vi "UHR-Fleezers Control (host) - 16.2.2v2.vi"() -> ()   [LabVIEW 2014] (continued)
        "Overflow (data lost)" <- TRUE ("Overflow (data lost)")
      }
    }
    n3205 = Build Array(w4581, w4580) -> (w4579:dbl[][])
    n3206 = To Double Precision Float(number=w4672) -> (double precision float=w4673:dbl[][])
    n3207 = feedback #8 "APD3"(w4368) -> (w4387:dbl[])
    n3208 = feedback #9 "APD2"(w4370) -> (w4602:dbl[])
    n3209 = feedback #10 "APD1"(w4372) -> (w4671:dbl[])
    n3210 = Build Array (concatenate)(w4387, w4368) -> (w4386:dbl[])
    n3211 = Build Array (concatenate)(w4602, w4370) -> (w4601:dbl[])
    n3212 = Build Array (concatenate)(w4671, w4372) -> (w4668:dbl[])
    n3213 = for {
      tunnel: w4370 -> [w4855] mode=indexing
      n3214 = call "Smart Buffer (DBL) 2.vi"("new element [write]"=w4855, "mode"=T26."write") -> ()  [unwired: 4 in, 6 out]
    }
    n3215 = Array Size(array=w4668) -> (size(s)=w4665:i32)
    n3216 = Array Size(array=w4372) -> (size(s)=w4667:i32)
    n3217 = Multiply(x=w4667, y="APD Ave N") -> (x*y=w4666:dbl)
    n3218 = Greater?(x=w4665, y=w4666) -> (0:w4669:bool)
    n3219 = Bundle("APD 1", "APD 2", "APD 3") -> (w4703:cluster{string, string, string})  [unwired: 1 out]
    n3220 = local read "Trap Sets"() -> (w4636:u32)
    n3221 = case shown="True" w4669 {
      tunnel: w4668 -> [w5112 w5121]
      tunnel: [w5112 w5119] -> w4643
      tunnel: w4666 -> [_ w5114]
      tunnel: w4665 -> [_ w5120]
      tunnel: w4601 -> [w5111 w5118]
      tunnel: [w5111 w5117] -> w4599
      tunnel: w4386 -> [w5110 w5116]
      tunnel: [w5110 w5113] -> w4449
      frame False {
      }
      frame True {
        n3222 = Subtract(x=w5120, y=w5114) -> (x-y=w5115:dbl)
        n3223 = Array Subset "APD3"(array=w5116, index=w5115, length=w5114) -> (w5113:dbl[])
        n3224 = Array Subset "APD2"(array=w5118, index=w5115, length=w5114) -> (w5117:dbl[])
        n3225 = Array Subset "APD1"(array=w5121, index=w5115, length=w5114) -> (w5119:dbl[])
      }
    }
    n3226 = feedback-in #8(w4449) -> ()
    n3227 = feedback-in #9(w4599) -> ()
    n3228 = feedback-in #10(w4643) -> ()
    n3229 = Cluster To Array(cluster=w4703) -> (array=w4700:string[])
    n3230 = for "APD" {
      tunnel: w4673 -> [w5368] mode=indexing
      tunnel: w4366 -> [w5375]
      tunnel: [w5371] -> w4603 mode=indexing
      tunnel: "APD Disp. Scale" -> [w5372]
      tunnel: w4700 -> [w5370] mode=indexing
      tunnel: "APD Disp. Downsample" -> [w5366]
      tunnel: [w5369] -> w4699
      workers-P: _ -> [_]
      tunnel: w4575 -> [w5365]
      n3231 = call "integrate 1D array interval - double.vi"("Ave N"=w5366, "Array In"=w5368) -> ("Array Out"=w5367:dbl[])  [unwired: 1 out]
      n3232 = Multiply(x=w5375, y=w5366) -> (x*y=w5369:dbl)
      n3233 = Divide(x=w5367, y=w5372) -> (x/y=w5373:dbl[])
      n3234 = Bundle By Name("t0"=w5365, "Y"=w5373, "dt"=w5369) -> (w5374:waveform(dbl))  [unwired: 1 out]
      n3235 = Set Waveform Attribute(5:w5370, 6:"NI_ChannelName" ("name"), 7:w5374) -> (3:w5371:waveform(dbl))  [unwired: 1 in, 2 out]
    }
    "APD Display Period (s)" <- w4699
    n3236 = Reciprocal(x=w4699) -> (1/x=→"APD Display Freq. (Hz)":dbl)
    n3237 = case "Deinterlace trap data, average down PSD" shown="2" w4636 {
      tunnel: w4548 -> [w5393 w5458]
      tunnel: [w5390 w5455] -> w4631
      tunnel: [w5393 w5457] -> w4539
      tunnel: "Detector Type" -> [w5392 w5453]
      tunnel: [w5391 w5456] -> w4630
      tunnel: [w5389 w5454] -> w4707
      frame 1, Default {
        n3238 = Divide(x=w5393, y=3276.7) -> (x/y=w5394:dbl[])
        n3239 = Decimate 1D Array(w5394) -> (w5403:dbl[], w5402:dbl[], w5401:dbl[], w5400:dbl[], w5399:dbl[], w5398:dbl[], w5397:dbl[], w5396:dbl[])
        n3240 = case shown="\"IR-QPD + PSD + FB-QPD position\"" w5392 {
          tunnel: w5403 -> [w5427 w5452]
          tunnel: w5402 -> [w5426 w5451]
          tunnel: w5401 -> [w5411 w5429]
          tunnel: w5400 -> [w5412 w5439]
          tunnel: w5399 -> [w5425 w5450]
          tunnel: w5398 -> [w5424 w5449]
          tunnel: w5397 -> [w5408 w5430]
          tunnel: w5396 -> [w5407 w5428]
          tunnel: [w5406 w5436] -> w5391
          tunnel: [w5405 w5435] -> w5390
          tunnel: [w5404 w5434] -> w5389
          frame "IR-QPD + PSD + FB-QPD", Default {
            w5404 = 0  # Channel pattern
            n3241 = Divide(x=w5427, y=w5412) -> (x/y=w5414:dbl[])
            n3242 = Divide(x=w5426, y=w5412) -> (x/y=w5413:dbl[])
            n3243 = Divide(x=w5425, y=w5408) -> (x/y=w5410:dbl[])
            n3244 = Divide(x=w5424, y=w5407) -> (x/y=w5409:dbl[])
            n3245 = Build Array(w5414, w5413, w5412, w5411, w5410, w5409, w5408, w5407) -> (w5405:dbl[][])
            n3246 = Bundle("T1 Y", "T1 X", "T1 Sum", "FB Sum", "PSD Y", "PSD X", "PSD Y Sum", "PSD X Sum") -> (w5423:T53)  [unwired: 1 out]
            n3247 = Cluster To Array(cluster=w5423) -> (array=w5406:string[])
          }
          frame "IR-QPD + PSD + FB-QPD position" {
            w5434 = 3  # Channel pattern
            n3248 = Negate(x=w5430) -> (-x=w5431:dbl[])
            n3249 = Divide(x=w5452, y=w5439) -> (x/y=w5441:dbl[])
            n3250 = Divide(x=w5451, y=w5439) -> (x/y=w5440:dbl[])
            n3251 = Divide(x=w5450, y=w5430) -> (x/y=w5438:dbl[])
            n3252 = Divide(x=w5449, y=w5431) -> (x/y=w5437:dbl[])
            n3253 = Build Array(w5441, w5440, w5439, w5428, w5429, w5438, w5437, w5430) -> (w5435:dbl[][])
            n3254 = Bundle("T1 Y", "T1 X", "T1 Sum", "FB X", "FB Sum", "PSD Y", "PSD X", "PSD Y Sum") -> (w5448:T53)  [unwired: 1 out]
            n3255 = Cluster To Array(cluster=w5448) -> (array=w5436:string[])
          }
        }
      }
      frame 2 {
        n3256 = case shown="\"IR-QPD + PSD + FB-QPD X position\", Default" w5453 {
          tunnel: w5458 -> [w5520 w5592 w5663]
          tunnel: [w5459 w5583 w5594] -> w5457
          tunnel: [w5486 w5574 w5641] -> w5456
          tunnel: [w5485 w5537 w5608] -> w5455
          tunnel: [w5479 w5572 w5639] -> w5454
          frame "IR-QPD + PSD + FB-QPD" {
            w5479 = 1  # Channel pattern
            # "time average x2 the 4th signal and the 4 psd signals (detection laser)"
            # "deinterlace 3 signals from qpd"
            n3257 = Decimate 1D Array(w5520) -> (w5519:i16[], w5518:i16[], w5484:i16[], w5517:i16[], w5507:i16[], w5505:i16[], w5504:i16[], w5502:i16[])
            n3258 = Decimate 1D Array(w5484) -> (w5483:i16[], w5482:i16[])
            n3259 = Decimate 1D Array(w5519) -> (w5516:i16[], w5488:i16[])
            n3260 = Decimate 1D Array(w5518) -> (w5515:i16[], w5513:i16[])
            n3261 = Decimate 1D Array(w5517) -> (w5514:i16[], w5512:i16[])
            n3262 = call "downsample 1D array - double.vi"("Ave N"=2.0, "Array In"=w5507) -> ("Array Out"=w5506:dbl[])  [unwired: 1 out]
            n3263 = call "downsample 1D array - double.vi"("Ave N"=2.0, "Array In"=w5505) -> ("Array Out"=w5487:dbl[])  [unwired: 1 out]
            n3264 = call "downsample 1D array - double.vi"("Ave N"=2.0, "Array In"=w5504) -> ("Array Out"=w5503:dbl[])  [unwired: 1 out]
            n3265 = call "downsample 1D array - double.vi"("Ave N"=2.0, "Array In"=w5502) -> ("Array Out"=w5501:dbl[])  [unwired: 1 out]
            n3266 = Interleave 1D Arrays(w5516, w5515, w5514, w5488, w5513, w5512, w5483, w5482, w5506, w5487, w5503, w5501) -> (w5500:dbl[])
            n3267 = Divide(x=w5500, y=3276.7) -> (x/y=w5499:dbl[])
            n3268 = Decimate 1D Array(w5499) -> (w5498:dbl[], w5497:dbl[], w5496:dbl[], w5495:dbl[], w5494:dbl[], w5493:dbl[], w5481:dbl[], w5480:dbl[], w5492:dbl[], w5491:dbl[], w5490:dbl[], w5489:dbl[])
            n3269 = Divide(x=w5498, y=w5496) -> (x/y=w5466:dbl[])
            n3270 = Divide(x=w5497, y=w5496) -> (x/y=w5465:dbl[])
            n3271 = Divide(x=w5495, y=w5493) -> (x/y=w5464:dbl[])
            n3272 = Divide(x=w5494, y=w5493) -> (x/y=w5463:dbl[])
            n3273 = Divide(x=w5492, y=w5490) -> (x/y=w5462:dbl[])
            n3274 = Divide(x=w5491, y=w5489) -> (x/y=w5461:dbl[])
            n3275 = Build Array(w5466, w5465, w5496, w5464, w5463, w5493, w5481, w5480, w5462, w5461, w5490, w5489) -> (w5485:dbl[][])
            n3276 = Bundle("T1 Y", "T1 X", "T1 Sum", "T2 Y", "T2 X", "T2 Sum", "T1 FB Sum", "T2 FB Sum", "PSD Y", "PSD X", "PSD Y Sum", "PSD X Sum") -> (w5467:T54)  [unwired: 1 out]
            n3277 = To Word Integer(number=w5500) -> (16bit integer=w5459:i16[])
            n3278 = Cluster To Array(cluster=w5467) -> (array=w5486:string[])
          }
          frame "IR-QPD + PSD + FB-QPD X position", Default {
            w5572 = 2  # Channel pattern
            # "time average x2 the 3 psd signals (detection laser)"
            # "deinterlace 3 signals from qpds"
            n3279 = Decimate 1D Array(w5592) -> (w5591:i16[], w5590:i16[], w5573:i16[], w5589:i16[], w5535:i16[], w5532:i16[], w5529:i16[], w5560:i16[])
            n3280 = Select(t=i16 -1, s="Flip X Sign", f=i16 1) -> (s? t:f=w5525:i16)
            n3281 = Multiply(x=w5590, y=w5525) -> (x*y=w5526:i16[])
            n3282 = Decimate 1D Array(w5573) -> (w5558:i16[], w5556:i16[])
            n3283 = Decimate 1D Array(w5591) -> (w5588:i16[], w5575:i16[])
            n3284 = Decimate 1D Array(w5526) -> (w5587:i16[], w5585:i16[])
            n3285 = Decimate 1D Array(w5589) -> (w5586:i16[], w5584:i16[])
            n3286 = Decimate 1D Array(w5560) -> (w5559:i16[], w5557:i16[])
            n3287 = call "downsample 1D array - I16.vi"("Ave N"=2.0, "Array In"=w5535) -> ("Array Out"=w5533:i16[])  [unwired: 1 in]
            n3288 = call "downsample 1D array - I16.vi"("Ave N"=2.0, "Array In"=w5529) -> ("Array Out"=w5527:i16[])  [unwired: 1 in]
            n3289 = call "downsample 1D array - I16.vi"("Ave N"=2.0, "Array In"=w5532) -> ("Array Out"=w5530:i16[])  [unwired: 1 in]
            n3290 = Interleave 1D Arrays(w5588, w5587, w5586, w5575, w5585, w5584, w5559, w5558, w5557, w5556, w5533, w5530, w5527) -> (w5583:i16[])
            n3291 = Divide(x=w5583, y=3276.7) -> (x/y=w5582:dbl[])
            n3292 = Decimate 1D Array(w5582) -> (w5581:dbl[], w5580:dbl[], w5579:dbl[], w5578:dbl[], w5577:dbl[], w5576:dbl[], w5548:dbl[], w5546:dbl[], w5545:dbl[], w5543:dbl[], w5542:dbl[], w5541:dbl[], w5538:dbl[])
            n3293 = Negate(x=w5538) -> (-x=w5536:dbl[])
            n3294 = Divide(x=w5542, y=w5538) -> (x/y=w5540:dbl[])
            n3295 = Divide(x=w5541, y=w5536) -> (x/y=w5539:dbl[])
            n3296 = Divide(x=w5581, y=w5579) -> (x/y=w5564:dbl[])
            n3297 = Divide(x=w5580, y=w5579) -> (x/y=w5563:dbl[])
            n3298 = Divide(x=w5578, y=w5576) -> (x/y=w5562:dbl[])
            n3299 = Divide(x=w5577, y=w5576) -> (x/y=w5561:dbl[])
            n3300 = Divide(x=w5548, y=w5546) -> (x/y=w5547:dbl[])
            n3301 = Divide(x=w5545, y=w5543) -> (x/y=w5544:dbl[])
            n3302 = Build Array(w5564, w5563, w5579, w5562, w5561, w5576, w5547, w5546, w5544, w5543, w5540, w5539, w5538) -> (w5537:dbl[][])
            n3303 = Bundle("T1 Y", "T1 X", "T1 Sum", "T2 Y", "T2 X", "T2 Sum", "T1 FB X", "T1 FB Sum", "T2 FB X", "T2 FB Sum", "PSD Y", "PSD X", "PSD Y Sum") -> (w5565:T55)  [unwired: 1 out]
            n3304 = Cluster To Array(cluster=w5565) -> (array=w5574:string[])
          }
          frame "IR-QPD + PSD + FB-QPD XY positions" {
            w5639 = 4  # Channel pattern
            # "time average x2 the 3 psd signals (detection laser)"
            # "deinterlace 3 signals from qpds"
            n3305 = Decimate 1D Array(w5663) -> (w5662:i16[], w5661:i16[], w5640:i16[], w5660:i16[], w5606:i16[], w5652:i16[], w5651:i16[], w5628:i16[])
            n3306 = Decimate 1D Array "Feedback Sum"(w5640) -> (w5624:i16[], w5622:i16[])
            n3307 = Decimate 1D Array "QPD Y"(w5662) -> (w5659:i16[], w5642:i16[])
            n3308 = Decimate 1D Array "QPD X"(w5661) -> (w5658:i16[], w5656:i16[])
            n3309 = Decimate 1D Array "Feedback Y"(w5606) -> (w5605:i16[], w5604:i16[])
            n3310 = Decimate 1D Array "QPD Sum"(w5660) -> (w5657:i16[], w5655:i16[])
            n3311 = Decimate 1D Array "Feedback X"(w5628) -> (w5625:i16[], w5623:i16[])
            n3312 = call "downsample 1D array - double.vi"("Ave N"=2.0, "Array In"=w5652) -> ("Array Out"=w5627:dbl[])  [unwired: 1 out]
            n3313 = call "downsample 1D array - double.vi"("Ave N"=2.0, "Array In"=w5651) -> ("Array Out"=w5626:dbl[])  [unwired: 1 out]
            n3314 = Interleave 1D Arrays(w5659, w5658, w5657, w5642, w5656, w5655, w5605, w5625, w5624, w5604, w5623, w5622, w5627, w5626) -> (w5650:dbl[])
            n3315 = Divide(x=w5650, y=3276.7) -> (x/y=w5649:dbl[])
            n3316 = Decimate 1D Array(w5649) -> (w5648:dbl[], w5647:dbl[], w5646:dbl[], w5645:dbl[], w5644:dbl[], w5643:dbl[], w5601:dbl[], w5615:dbl[], w5599:dbl[], w5600:dbl[], w5613:dbl[], w5597:dbl[], w5611:dbl[], w5609:dbl[])
            n3317 = Negate(x=w5609) -> (-x=w5607:dbl[])
            n3318 = Divide(x=w5611, y=w5607) -> (x/y=w5610:dbl[])
            n3319 = Divide(x=w5600, y=w5597) -> (x/y=w5596:dbl[])
            n3320 = Divide(x=w5601, y=w5599) -> (x/y=w5598:dbl[])
            n3321 = Divide(x=w5648, y=w5646) -> (x/y=w5632:dbl[])
            n3322 = Divide(x=w5647, y=w5646) -> (x/y=w5631:dbl[])
            n3323 = Divide(x=w5645, y=w5643) -> (x/y=w5630:dbl[])
            n3324 = Divide(x=w5644, y=w5643) -> (x/y=w5629:dbl[])
            n3325 = Divide(x=w5615, y=w5599) -> (x/y=w5614:dbl[])
            n3326 = Divide(x=w5613, y=w5597) -> (x/y=w5612:dbl[])
            n3327 = Build Array(w5632, w5631, w5646, w5630, w5629, w5643, w5598, w5614, w5599, w5596, w5612, w5597, w5610, w5609) -> (w5608:dbl[][])
            n3328 = Bundle("T1 Y", "T1 X", "T1 Sum", "T2 Y", "T2 X", "T2 Sum", "T1 FB Y", "T1 FB X", "T1 FB Sum", "T2 FB Y", "T2 FB X", "T2 FB Sum", "PSD X", "PSD Y Sum") -> (w5595:T56)  [unwired: 1 out]
            n3329 = To Word Integer(number=w5650) -> (16bit integer=w5594:i16[])
            n3330 = Cluster To Array(cluster=w5595) -> (array=w5641:string[])
          }
        }
      }
    }
    "AI labels" <- w4630
    n3331 = Array Size(array=w4643) -> (size(s)=w4664:i32)
    n3332 = call <vilib>:"Std Deviation and Variance.vi"("X"=w4599) -> ("standard deviation"=w4598:dbl)  [unwired: 1 in, 2 out]
    n3333 = Add Array Elements(numeric array=w4599) -> (sum=w4600:dbl)
    n3334 = Add Array Elements(numeric array=w4643) -> (sum=w4674:dbl)
    n3335 = call <vilib>:"Std Deviation and Variance.vi"("X"=w4643) -> ("standard deviation"=w4642:dbl)  [unwired: 1 in, 2 out]
    n3336 = Divide(x=w4598, y=w4366) -> (x/y=w4595:dbl)
    "Rate sigma (Hz) 2" <- w4595
    n3337 = Multiply(x=w4366, y=w4664) -> (x*y=w4450:dbl)
    "Int. Time (s)" <- w4450
    n3338 = Divide(x=w4600, y=w4450) -> (x/y=w4596:dbl)
    "APD 2 Rate (Hz)" <- w4596
    n3339 = Multiply(x="APD Disp. Scale", y=w4603) -> (x*y=w4609:waveform(dbl)[])
    n3340 = Divide(x=w4674, y=w4450) -> (x/y=w4640:dbl)
    "APD 1 Rate (Hz)" <- w4640
    n3341 = Divide(x=w4642, y=w4366) -> (x/y=w4641:dbl)
    "Rate sigma (Hz)" <- w4641
    n3342 = Divide(x=w4595, y=w4596) -> (x/y=→"Sigma/Mean 2":dbl)
    n3343 = Multiply(x="APD Disp. Downsample", y=w4366) -> (x*y=w4606:dbl)
    n3344 = Divide(x=w4641, y=w4640) -> (x/y=→"Sigma/Mean":dbl)
    n3345 = Divide(x=w4609, y=w4606) -> (x/y=w4441:waveform(dbl)[])
    n3346 = Index Array(array=w4441, index=0) -> (element=w4592:waveform(dbl))
    n3347 = Index Array(array=w4441, index=1) -> (element=w4590:waveform(dbl))
    n3348 = Index Array(array=w4441, index=2) -> (element=w4443:waveform(dbl))
    n3349 = Subtract(x=w4592, y="APD 1 Offset") -> (x-y=w4588:waveform(dbl))
    n3350 = Subtract(x=w4590, y="APD 2 Offset") -> (x-y=w4587:waveform(dbl))
    n3351 = Subtract(x=w4443, y="APD 3 Offset") -> (x-y=w4440:waveform(dbl))
    n3352 = Add Array Elements(numeric array=w4449) -> (sum=w4452:dbl)
    n3353 = call <vilib>:"Std Deviation and Variance.vi"("X"=w4449) -> ("standard deviation"=w4451:dbl)  [unwired: 1 in, 2 out]
    n3354 = Build Array(w4588, w4587, w4440) -> (→"APD Chart":waveform(dbl)[])
    n3355 = Divide(x=w4452, y=w4450) -> (x/y=w4447:dbl)
    "APD 3 Rate (Hz)" <- w4447
    n3356 = Divide(x=w4451, y=w4366) -> (x/y=w4448:dbl)
    "Rate sigma (Hz) 3" <- w4448
    n3357 = Divide(x=w4448, y=w4447) -> (x/y=→"Sigma/Mean 3":dbl)
    n3358 = local read "Data Period (s)"() -> (w4498:dbl)
    n3359 = local read "BD 1 Frequency 2 (MHz)"() -> (w4531:dbl)
    n3360 = local read "BD 1 Frequency 1 (MHz)"() -> (w4532:dbl)
    n3361 = Decimate 1D Array(w4539) -> (w4563:i16[], w4562:i16[], w4560:i16[], w4559:i16[])  [unwired: 9 out]
    n3362 = Multiply(x=w4498, y="Trap Pos. Disp. Downsample") -> (x*y=w4496:dbl)
    n3363 = Divide(x=w4563, y=w4562) -> (x/y=w4564:dbl[])
    n3364 = Divide(x=w4560, y=w4559) -> (x/y=w4561:dbl[])
    n3365 = local read "AOM X Cal (nm/MHz)"() -> (w4529:dbl)
    n3366 = Split 1D Array(array=w4564, index="N El. to Ave.") -> (second subarray=w4567:dbl[])  [unwired: 1 out]
    n3367 = Split 1D Array(array=w4561, index="N El. to Ave.") -> (second subarray=w4566:dbl[])  [unwired: 1 out]
    n3368 = Multiply(x=w4498, y="Trap Disp. Downsample") -> (x*y=w4577:dbl)
    "Display Period (s)" <- w4577
    n3369 = for "Trap AI" {
      tunnel: [w5388] -> w4410 mode=indexing
      tunnel: w4575 -> [w5379]
      tunnel: "Trap Disp. Downsample" -> [w5386]
      tunnel: w4631 -> [w5384] mode=indexing
      tunnel: w4498 -> [w5383]
      tunnel: w4630 -> [w5382] mode=indexing
      tunnel: [w5381] -> w4605 mode=indexing
      tunnel: w4577 -> [w5380]
      workers-P: _ -> [_]
      n3370 = Bundle By Name("Y"=w5384, "dt"=w5383) -> (w5385:waveform(dbl))  [unwired: 1 out]
      n3371 = Set Waveform Attribute(5:w5382, 6:"NI_ChannelName" ("name"), 7:w5385) -> (3:w5381:waveform(dbl))  [unwired: 1 in, 2 out]
      n3372 = call "downsample 1D array - double.vi"("Ave N"=w5386, "Array In"=w5384) -> ("Array Out"=w5387:dbl[])  [unwired: 1 out]
      n3373 = Bundle By Name(cluster=w5381, "t0"=w5379, "Y"=w5387, "dt"=w5380) -> (w5388:waveform(dbl))
    }
    n3374 = Bundle("BD 1 Frequency 1 (MHz)"=w4532, "BD 1 Frequency 2 (MHz)"=w4531) -> (w4533:T57)  [unwired: 1 out]
    n3375 = call-poly <vilib>:"Mean.vi"("X"=w4566) -> ("mean"=w4554:dbl)  [unwired: 1 out]
    n3376 = call-poly <vilib>:"Mean.vi"("X"=w4567) -> ("mean"=w4555:dbl)  [unwired: 1 out]
    n3377 = Reciprocal(x=w4577) -> (1/x=→"Trap Disp. Freq. (Hz)":dbl)
    n3378 = Cluster To Array(cluster=w4533) -> (array=w4530:dbl[])
    n3379 = local read "Trap X AI1 (DMA)"() -> (w4565:T15)
    n3380 = local read "Data points/scans (MCL)"() -> (w4684:dbl)
    n3381 = To Fixed-Point(number=w4554) -> (fixed-point=w4552:fxp<+/-,16,1>)  [unwired: 1 in]
    n3382 = To Fixed-Point(number=w4555) -> (fixed-point=w4553:fxp<+/-,16,1>)  [unwired: 1 in]
    n3383 = Bundle("Trap 1 Pos.", "Trap 2 Pos.") -> (w4574:cluster{string, string})  [unwired: 1 out]
    n3384 = Bundle By Name(cluster=w4565, "Set 1"=w4553, "Set 2"=w4552) -> (→"Trap X AI1 (DMA)":T15)
    n3385 = Cluster To Array(cluster=w4574) -> (array=w4571:string[])
    n3386 = Unbundle(w4438) -> ("Array Out"=w4439:dbl[])  [unwired: 2 out]
    n3387 = Select(t=-1.0, s="Negate Y Axis", f=1.0) -> (s? t:f=w4515:dbl)
    n3388 = for "Trap Position" {
      tunnel: w4579 -> [w5026] mode=indexing
      tunnel: "Trap Pos. Disp. Downsample" -> [w5025]
      tunnel: w4496 -> [w5023]
      tunnel: w4575 -> [w5022]
      tunnel: w4571 -> [w5020] mode=indexing
      tunnel: [w5019] -> w4485 mode=indexing
      tunnel: w4530 -> [w5017] mode=indexing
      tunnel: w4529 -> [w5015]
      tunnel: w4515 -> [w5014]
      n3389 = call "downsample 1D array - double.vi"("Ave N"=w5025, "Array In"=w5026) -> ("Array Out"=w5024:dbl[])  [unwired: 1 out]
      n3390 = Subtract(x=w5024, y=w5017) -> (x-y=w5018:dbl[])
      n3391 = Multiply(x=w5015, y=w5018) -> (x*y=w5016:dbl[])
      n3392 = Multiply(x=w5014, y=w5016) -> (x*y=w5013:dbl[])
      n3393 = Bundle By Name("Y"=w5013, "dt"=w5023, "t0"=w5022) -> (w5021:waveform(dbl))  [unwired: 1 out]
      n3394 = Set Waveform Attribute(5:w5020, 6:"NI_ChannelName" ("name"), 7:w5021) -> (3:w5019:waveform(dbl))  [unwired: 1 in, 2 out]
    }
    n3395 = To Double Precision Float(number=w4439) -> (double precision float=w4628:dbl[])
    n3396 = local read "Display Period (s)"() -> (w4619:dbl)
    n3397 = Increment(x=w4684) -> (x+1=w4685:dbl)
    n3398 = Index Array(array=w4485, index=0) -> (element=w4489:waveform(dbl))
    n3399 = Index Array(array=w4485, index=1) -> (element=w4484:waveform(dbl))
    n3400 = feedback #11(w4685) -> (w4688:dbl)
    n3401 = Select(t=0, s=w4675, f=w4688) -> (s? t:f=w4681:dbl)
    n3402 = Array Size(array=w4628) -> (size(s)=w4687:i32)
    n3403 = Add(x=w4687, y=w4681) -> (x+y=w4682:dbl)
    n3404 = Unbundle By Name(w4489) -> ("Y"=w4490:dbl[])
    n3405 = Divide(x="Bead Sep. Int. Time (s)", y=w4619) -> (x/y=w4525:dbl)
    n3406 = Add(x=w4490, y="FB Trap Pos Offset") -> (x+y=w4488:dbl[])
    "T1 x pos data" <- w4488
    n3407 = Greater?(x=w4682, y=w4684) -> (0:w4683:bool)
    n3408 = feedback #12(w4488) -> (w4527:dbl[])
    n3409 = Build Array (concatenate)(w4488, w4527) -> (w4526:dbl[])
    n3410 = Bundle By Name(cluster=w4489, "Y"=w4488) -> (w4487:waveform(dbl))
    n3411 = Select(t=w4681, s=w4683, f=w4682) -> (s? t:f=w4680:dbl)
    n3412 = feedback-in #11(w4680) -> ()
    n3413 = local read "MCL Scanning"() -> (w4678:bool)
    n3414 = Bundle(w4487, w4484) -> (w4483:cluster{waveform(dbl), waveform(dbl)})  [unwired: 1 out]
    n3415 = Index Array(array=w4410, index="index 1") -> (element=w4432:waveform(dbl))
    n3416 = Index Array(array=w4410, index="index 2") -> (element=w4436:waveform(dbl))
    n3417 = Split 1D Array(array=w4526, index=w4525) -> (first subarray=w4519:dbl[])  [unwired: 1 out]
    n3418 = feedback-in #12(w4519) -> ()
    n3419 = Unbundle By Name(w4432) -> ("Y"=w4431:dbl[])
    n3420 = Unbundle By Name(w4436) -> ("Y"=w4435:dbl[])
    n3421 = Not(x=w4683) -> (.not. x?=w4677:bool)
    n3422 = Cluster To Array(cluster=w4483) -> (array=w4462:waveform(dbl)[])
    "Trap Positions" <- w4462
    n3423 = call-poly <vilib>:"Mean.vi"("X"=w4519) -> ("mean"=w4518:dbl)  [unwired: 1 out]
    "Mean T1 Position (nm)" <- w4518
    n3424 = Subtract(x=w4519, y=w4518) -> (x-y=w4524:dbl[])
    n3425 = Square(x=w4524) -> (x^2=w4523:dbl[])
    n3426 = And(x=w4677, y=w4678) -> (x .and. y?=w4679:bool)
    n3427 = call-poly <vilib>:"Mean.vi"("X"=w4523) -> ("mean"=w4522:dbl)  [unwired: 1 out]
    n3428 = call-poly <vilib>:"Mean.vi"("X"=w4431) -> ("mean"=→"Trap 1 sum mean":dbl)  [unwired: 1 out]
    n3429 = call-poly <vilib>:"Mean.vi"("X"=w4435) -> ("mean"=→"Trap 2 sum mean":dbl)  [unwired: 1 out]
    n3430 = Square Root(x=w4522) -> (sqrt(x)=w4521:dbl)
    n3431 = Or(x=w4679, y=w4675) -> (x .or. y?=w4676:bool)
    n3432 = Build Array (concatenate)(w4603, w4410) -> (w4390:waveform(dbl)[])
    "All Signals" <- w4390
    n3433 = Equal?(x="Tab Control 6", y=T45."High Res Display") -> (x = y?=w4632:bool)
    n3434 = case shown="False" "X or Y?" {
      tunnel: w4410 -> [w4845 w4851]
      tunnel: [w4846 w4850] -> w4405
      tunnel: [w4844 w4849] -> w4402
      frame False {
        n3435 = Index Array(array=w4845, index=0) -> (element=w4846:waveform(dbl))
        n3436 = Index Array(array=w4845, index=3) -> (element=w4844:waveform(dbl))
      }
      frame True {
        n3437 = Index Array(array=w4851, index=1) -> (element=w4850:waveform(dbl))
        n3438 = Index Array(array=w4851, index=4) -> (element=w4849:waveform(dbl))
      }
    }
    n3439 = Multiply(x=10.0, y=w4521) -> (x*y=→"Trap 1 Position RMS (A)":dbl)
    n3440 = case "For displaying the high resolution display (no downsampling)" shown="True" w4632 {
      tunnel: w4605 -> [_ w5046]
      frame False {
      }
      frame True {
        n3441 = Index Array(array=w5046, index="High Res. Display") -> (element=w5047:waveform(dbl))
        n3442 = call <vilib>:"Std Deviation and Variance.vi"("X"=w5047) -> ("mean"=w5054:dbl, "standard deviation"=w5059:dbl)  [unwired: 1 in, 1 out]
        "Mean Intensity" <- w5054
        "Sigma" <- w5059
        n3443 = Subtract(x=w5047, y=w5054) -> (x-y=w5053:waveform(dbl))
        n3444 = Select(t=w5053, s="Subtract mean", f=w5047) -> (s? t:f=→"1 Channel":waveform(dbl))
        n3445 = Divide(x=w5059, y=w5054) -> (x/y=→"Sigma/Mean":dbl)
        n3446 = feedback #13(1) -> (w5048:i32)
        n3447 = Greater Or Equal?(x=w5048, y="Slow mean N ave.") -> (x >= y?=w5061:bool)
        n3448 = Increment(x=w5048) -> (x+1=w5063:i32)
        n3449 = Select(t=1, s=w5061, f=w5063) -> (s? t:f=w5050:i32)
        n3450 = feedback-in #13(w5050) -> ()
        n3451 = feedback #14() -> (w5051:waveform(dbl))  [unwired: 1 out]
        n3452 = case shown="Default" w5048 {
          tunnel: [w5066 w5069] -> w5052
          tunnel: w5051 -> [w5068 _]
          tunnel: w5047 -> [w5067 w5069]
          frame Default {
            n3453 = call-poly <vilib>:"Append Waveforms.vi"("waveform B"=w5067, "waveform A"=w5068) -> ("waveform out"=w5066:waveform(dbl))  [unwired: 1 in, 8 out]
          }
          frame 1 {
          }
        }
        n3454 = feedback-in #14(w5052) -> ()
        n3455 = case shown="True" w5061 {
          tunnel: w5052 -> [_ w5065]
          frame False {
          }
          frame True {
            n3456 = call-poly <vilib>:"Mean.vi"("X"=w5065) -> ("mean"=→"Slow mean":dbl)  [unwired: 1 out]
          }
        }
      }
    }
    n3457 = case "For plotting results of scanning MCL (fluorescence and detection laser images)" shown="True" w4676 {
      tunnel: w4675 -> [_ w5129]
      tunnel: w4684 -> [_ _]
      tunnel: w4605 -> [_ w5256]
      tunnel: w4585 -> [_ w5164]
      tunnel: w4438 -> [_ w5135]
      frame False {
      }
      frame True {
        w5145 = u32 0 items=["Horizontal", "Vertical", "Central", "1st Diagonal", "2nd Diagonal"] ("Type of Symmetry")
        w5171 = u32 0 items=["Horizontal", "Vertical", "Central", "1st Diagonal", "2nd Diagonal"] ("Type of Symmetry")
        w5195 = u32 0 items=["Horizontal", "Vertical", "Central", "1st Diagonal", "2nd Diagonal"] ("Type of Symmetry")
        w5198 = u32 0 items=["Horizontal", "Vertical", "Central", "1st Diagonal", "2nd Diagonal"] ("Type of Symmetry")
        w5227 = u32 0 items=["Horizontal", "Vertical", "Central", "1st Diagonal", "2nd Diagonal"] ("Type of Symmetry")
        n3458 = Unbundle(w5135) -> ("Array Out"=w5134:dbl[], "Array Out"=w5132:dbl[], "Array Out"=w5130:dbl[])
        n3459 = To Double Precision Float(number=w5134) -> (double precision float=w5133:dbl[])
        n3460 = To Double Precision Float(number=w5132) -> (double precision float=w5131:dbl[])
        n3461 = To Double Precision Float(number=w5130) -> (double precision float=w5123:dbl[])
        n3462 = Index Array(array=w5256, index=10) -> (element=w5262:waveform(dbl))
        n3463 = Index Array(array=w5256, index=11) -> (element=w5259:waveform(dbl))
        n3464 = local read "Cycles/step (MCL)"() -> (w5212:u64)
        n3465 = Index Array(array=w5256, index="Channel") -> (element=w5258:waveform(dbl))
        n3466 = Unbundle(w5164) -> ("New Image"=w5163:T2, "New Image"=w5162:T2, "New Image"=w5136:T2, "New Image"=w5137:T2, "New Image"=w5138:T2)
        n3467 = local read "Scan steps (MCL)"() -> (w5125:u64)
        n3468 = Unbundle By Name(w5262) -> ("Y"=w5214:dbl[])
        n3469 = Unbundle By Name(w5259) -> ("Y"=w5216:dbl[])
        n3470 = local read "Scan lines (y)"() -> (w5126:u64)
        n3471 = local read "N APD Samp/step"() -> (w5128:dbl)
        n3472 = Unbundle By Name(w5258) -> ("Y"=w5221:dbl[])
        n3473 = call "downsample 1D array - double.vi"("Ave N"=w5212, "Array In"=w5214) -> ("Array Out"=w5213:dbl[])  [unwired: 1 out]
        n3474 = call "downsample 1D array - double.vi"("Ave N"=w5212, "Array In"=w5216) -> ("Array Out"=w5215:dbl[])  [unwired: 1 out]
        n3475 = call "downsample 1D array - double.vi"("Ave N"=w5212, "Array In"=w5221) -> ("Array Out"=w5220:dbl[])  [unwired: 1 out]
        n3476 = Multiply(x=w5125, y=u64 2) -> (x*y=w5127:u64)
        n3477 = feedback #15(w5131) -> (w5189:dbl[])
        n3478 = Build Array (concatenate)(w5189, w5131) -> (w5188:dbl[])
        n3479 = feedback #16(w5123) -> (w5124:dbl[])
        n3480 = Build Array (concatenate)(w5124, w5123) -> (w5122:dbl[])
        n3481 = Select(t=w5131, s=w5129, f=w5188) -> (s? t:f=w5173:dbl[])
        n3482 = feedback-in #15(w5173) -> ()
        n3483 = Select(t=w5123, s=w5129, f=w5122) -> (s? t:f=w5147:dbl[])
        n3484 = feedback-in #16(w5147) -> ()
        n3485 = feedback #17(w5133) -> (w5282:dbl[])
        n3486 = Build Array (concatenate)(w5282, w5133) -> (w5264:dbl[])
        n3487 = Select(t=w5133, s=w5129, f=w5264) -> (s? t:f=w5268:dbl[])
        n3488 = feedback-in #17(w5268) -> ()
        n3489 = feedback #18(w5213) -> (w5270:dbl[])
        n3490 = Build Array (concatenate)(w5270, w5213) -> (w5261:dbl[])
        n3491 = feedback #19(w5220) -> (w5280:dbl[])
        n3492 = Build Array (concatenate)(w5280, w5220) -> (w5279:dbl[])
        n3493 = feedback #20(w5215) -> (w5272:dbl[])
        n3494 = Build Array (concatenate)(w5272, w5215) -> (w5273:dbl[])
        n3495 = Select(t=w5213, s=w5129, f=w5261) -> (s? t:f=w5217:dbl[])
        n3496 = feedback-in #18(w5217) -> ()
        n3497 = Select(t=w5220, s=w5129, f=w5279) -> (s? t:f=w5219:dbl[])
        n3498 = feedback-in #19(w5219) -> ()
        n3499 = Select(t=w5215, s=w5129, f=w5273) -> (s? t:f=w5218:dbl[])
        n3500 = feedback-in #20(w5218) -> ()
        n3501 = call "integrate 1D array interval - double.vi"("Ave N"=w5128, "Array In"=w5173) -> ("Array Out"=w5184:dbl[])  [unwired: 1 out]
        n3502 = call "integrate 1D array interval - double.vi"("Ave N"=w5128, "Array In"=w5147) -> ("Array Out"=w5158:dbl[])  [unwired: 1 out]
        n3503 = call "integrate 1D array interval - double.vi"("Ave N"=w5128, "Array In"=w5268) -> ("Array Out"=w5267:dbl[])  [unwired: 1 out]
        n3504 = Array Size(array=w5184) -> (size(s)=w5185:i32)
        n3505 = Array Size(array=w5158) -> (size(s)=w5159:i32)
        n3506 = Array Size(array=w5267) -> (size(s)=w5269:i32)
        n3507 = Multiply(x=w5126, y=w5127) -> (x*y=w5187:u64)
        n3508 = Multiply(x=w5126, y=w5127) -> (x*y=w5161:u64)
        n3509 = Multiply(x=w5126, y=w5127) -> (x*y=w5277:u64)
        n3510 = Subtract(x=w5187, y=w5185) -> (x-y=w5178:u64)
        n3511 = call-poly <vilib>:"Mean.vi"("X"=w5184) -> ("mean"=w5175:dbl)  [unwired: 1 out]
        n3512 = Subtract(x=w5161, y=w5159) -> (x-y=w5152:u64)
        n3513 = call-poly <vilib>:"Mean.vi"("X"=w5158) -> ("mean"=w5149:dbl)  [unwired: 1 out]
        n3514 = Subtract(x=w5277, y=w5269) -> (x-y=w5211:u64)
        n3515 = call-poly <vilib>:"Mean.vi"("X"=w5267) -> ("mean"=w5208:dbl)  [unwired: 1 out]
        n3516 = call-poly <vilib>:"Mean.vi"("X"=w5217) -> ("mean"=w5201:dbl)  [unwired: 1 out]
        n3517 = call-poly <vilib>:"Mean.vi"("X"=w5219) -> ("mean"=w5206:dbl)  [unwired: 1 out]
        n3518 = call-poly <vilib>:"Mean.vi"("X"=w5218) -> ("mean"=w5204:dbl)  [unwired: 1 out]
        n3519 = Initialize Array(1.0 ("element"), w5178) -> (w5174:dbl[])
        n3520 = Initialize Array(1.0 ("element"), w5152) -> (w5148:dbl[])
        n3521 = Initialize Array(1.0 ("element"), w5211) -> (w5202:dbl[])
        n3522 = Multiply(x=w5174, y=w5175) -> (x*y=w5176:dbl[])
        n3523 = Multiply(x=w5148, y=w5149) -> (x*y=w5150:dbl[])
        n3524 = Multiply(x=w5202, y=w5208) -> (x*y=w5209:dbl[])
        n3525 = Multiply(x=w5202, y=w5204) -> (x*y=w5205:dbl[])
        n3526 = Multiply(x=w5202, y=w5206) -> (x*y=w5207:dbl[])
        n3527 = Multiply(x=w5202, y=w5201) -> (x*y=w5203:dbl[])
        n3528 = Build Array (concatenate)(w5184, w5176) -> (w5186:dbl[])
        n3529 = Build Array (concatenate)(w5158, w5150) -> (w5160:dbl[])
        n3530 = Build Array (concatenate)(w5267, w5209) -> (w5276:dbl[])
        n3531 = Build Array (concatenate)(w5217, w5203) -> (w5271:dbl[])
        n3532 = Build Array (concatenate)(w5219, w5207) -> (w5275:dbl[])
        n3533 = Build Array (concatenate)(w5218, w5205) -> (w5274:dbl[])
        n3534 = Reshape Array(w5186, w5126, w5127) -> (w5182:dbl[][])
        n3535 = Reshape Array(w5160, w5126, w5127) -> (w5156:dbl[][])
        n3536 = Reshape Array(w5276, w5126, w5127) -> (w5254:dbl[][])
        n3537 = Reshape Array(w5271, w5126, w5127) -> (w5237:dbl[][])
        n3538 = Reshape Array(w5275, w5126, w5127) -> (w5229:dbl[][])
        n3539 = Reshape Array(w5274, w5126, w5127) -> (w5244:dbl[][])
        n3540 = Array Subset(array=w5182, index (col)=0 ("index"), length (col)=w5125) -> (w5181:dbl[][])  [unwired: 2 in]
        n3541 = Array Subset(array=w5182, index (col)=w5125) -> (w5179:dbl[][])  [unwired: 3 in]
        n3542 = Array Subset(array=w5156, index (col)=0 ("index"), length (col)=w5125) -> (w5155:dbl[][])  [unwired: 2 in]
        n3543 = Array Subset(array=w5156, index (col)=w5125) -> (w5153:dbl[][])  [unwired: 3 in]
        n3544 = Array Subset(array=w5244, index (col)=0 ("index"), length (col)=w5125) -> (w5249:dbl[][])  [unwired: 2 in]
        n3545 = Array Subset(array=w5244, index (col)=w5125) -> (w5247:dbl[][])  [unwired: 3 in]
        n3546 = Array Subset(array=w5254, index (col)=0 ("index"), length (col)=w5125) -> (w5253:dbl[][])  [unwired: 2 in]
        n3547 = Array Subset(array=w5254, index (col)=w5125) -> (w5251:dbl[][])  [unwired: 3 in]
        n3548 = Array Subset(array=w5229, index (col)=0 ("index"), length (col)=w5125) -> (w5235:dbl[][])  [unwired: 2 in]
        n3549 = Array Subset(array=w5229, index (col)=w5125) -> (w5233:dbl[][])  [unwired: 3 in]
        n3550 = Array Subset(array=w5237, index (col)=0 ("index"), length (col)=w5125) -> (w5242:dbl[][])  [unwired: 2 in]
        n3551 = Array Subset(array=w5237, index (col)=w5125) -> (w5240:dbl[][])  [unwired: 3 in]
        n3552 = for {
          tunnel: w5181 -> [w5286] mode=indexing
          tunnel: [w5285] -> w5180 mode=indexing
          workers-P: _ -> [_]
          n3553 = Reverse 1D Array(array=w5286) -> (reversed array=w5285:dbl[])
        }
        n3554 = for {
          tunnel: w5155 -> [w5284] mode=indexing
          tunnel: [w5283] -> w5154 mode=indexing
          workers-P: _ -> [_]
          n3555 = Reverse 1D Array(array=w5284) -> (reversed array=w5283:dbl[])
        }
        n3556 = for {
          tunnel: w5249 -> [w5292] mode=indexing
          tunnel: [w5291] -> w5248 mode=indexing
          workers-P: _ -> [_]
          n3557 = Reverse 1D Array(array=w5292) -> (reversed array=w5291:dbl[])
        }
        n3558 = for {
          tunnel: w5253 -> [w5294] mode=indexing
          tunnel: [w5293] -> w5252 mode=indexing
          workers-P: _ -> [_]
          n3559 = Reverse 1D Array(array=w5294) -> (reversed array=w5293:dbl[])
        }
        n3560 = for {
          tunnel: w5235 -> [w5288] mode=indexing
          tunnel: [w5287] -> w5234 mode=indexing
          workers-P: _ -> [_]
          n3561 = Reverse 1D Array(array=w5288) -> (reversed array=w5287:dbl[])
        }
        n3562 = for {
          tunnel: w5242 -> [w5290] mode=indexing
          tunnel: [w5289] -> w5241 mode=indexing
          workers-P: _ -> [_]
          n3563 = Reverse 1D Array(array=w5290) -> (reversed array=w5289:dbl[])
        }
        n3564 = Index Array(array=w5254, index (row)=0) -> (element=→"Waveform Graph":dbl[])  [unwired: 1 in]
        n3565 = Add(x=w5180, y=w5179) -> (x+y=w5166:dbl[][])
        n3566 = Add(x=w5154, y=w5153) -> (x+y=w5140:dbl[][])
        n3567 = Add(x=w5248, y=w5247) -> (x+y=w5246:dbl[][])
        n3568 = Add(x=w5252, y=w5251) -> (x+y=w5226:dbl[][])
        n3569 = Add(x=w5234, y=w5233) -> (x+y=w5232:dbl[][])
        n3570 = Add(x=w5241, y=w5240) -> (x+y=w5239:dbl[][])
        n3571 = Divide(x=w5232, y=2) -> (x/y=w5230:dbl[][])
        n3572 = Divide(x=w5246, y=2) -> (x/y=w5191:dbl[][])
        n3573 = To Single Precision Float(number=w5226) -> (single precision float=w5225:sgl[][])
        n3574 = To Single Precision Float(number=w5166) -> (single precision float=w5170:sgl[][])
        n3575 = To Single Precision Float(number=w5140) -> (single precision float=w5144:sgl[][])
        n3576 = Divide(x=w5239, y=2) -> (x/y=w5193:dbl[][])
        n3577 = Transpose 2D Array(2D array=w5230) -> (transposed array=→"Data map":dbl[][])
        n3578 = To Single Precision Float(number=w5191) -> (single precision float=w5197:sgl[][])
        n3579 = To Single Precision Float(number=w5193) -> (single precision float=w5194:sgl[][])
        n3580 = call "IMAQ ArrayToImage"("Image Pixels (Float)"=w5225, "Image"=w5163) -> ("Image Out"=w5228:T2)  [unwired: 8 in, 1 out]
        n3581 = call "IMAQ ArrayToImage"("Image Pixels (Float)"=w5170, "Image"=w5162) -> ("Image Out"=w5172:T2)  [unwired: 8 in, 1 out]
        n3582 = call "IMAQ ArrayToImage"("Image Pixels (Float)"=w5144, "Image"=w5136) -> ("Image Out"=w5146:T2)  [unwired: 8 in, 1 out]
        n3583 = call "IMAQ ArrayToImage"("Image Pixels (Float)"=w5197, "Image"=w5137) -> ("Image Out"=w5199:T2)  [unwired: 8 in, 1 out]
        n3584 = call "IMAQ Symmetry"("Type of Symmetry"=w5227, "Image Src"=w5228) -> ("Image Dst Out"=w5223:T2)  [unwired: 3 in, 1 out]
        n3585 = call "IMAQ ArrayToImage"("Image Pixels (Float)"=w5194, "Image"=w5138) -> ("Image Out"=w5196:T2)  [unwired: 8 in, 1 out]
        n3586 = call "IMAQ Symmetry"("Type of Symmetry"=w5171, "Image Src"=w5172) -> ("Image Dst Out"=w5168:T2)  [unwired: 3 in, 1 out]
        n3587 = call "IMAQ Symmetry"("Type of Symmetry"=w5145, "Image Src"=w5146) -> ("Image Dst Out"=w5142:T2)  [unwired: 3 in, 1 out]
        n3588 = call "IMAQ Symmetry"("Type of Symmetry"=w5198, "Image Src"=w5199) -> ("Image Dst Out"=→"Detection Laser X":T2)  [unwired: 3 in, 1 out]
        n3589 = call "IMAQ Symmetry"("Type of Symmetry"=w5195, "Image Src"=w5196) -> ("Image Dst Out"=→"Detection Laser Y":T2)  [unwired: 3 in, 1 out]
        n3590 = call "IMAQ Set Simple Calibration"("Calibration Axis Info"=T46 {"Origin Pixel"={"X"=0.0, "Y"=0.0}, "Angle Relative to Horizontal (deg)"=0.0, "Axis Reference"=0}, "Grid Descriptor"=T47 {"X Step"=0.3, "Y Step"=0.3, "Unit"=enum."Undefined"}, "Image"=w5223) -> ("Calibrated Image"=→"APD 1":T2)  [unwired: 7 in, 1 out]
        n3591 = call "IMAQ Set Simple Calibration"("Calibration Axis Info"=T46 {"Origin Pixel"={"X"=0.0, "Y"=0.0}, "Angle Relative to Horizontal (deg)"=0.0, "Axis Reference"=0}, "Grid Descriptor"=T47 {"X Step"=0.3, "Y Step"=0.3, "Unit"=enum."Undefined"}, "Image"=w5168) -> ("Calibrated Image"=→"APD 2":T2)  [unwired: 7 in, 1 out]
        n3592 = call "IMAQ Set Simple Calibration"("Calibration Axis Info"=T46 {"Origin Pixel"={"X"=0.0, "Y"=0.0}, "Angle Relative to Horizontal (deg)"=0.0, "Axis Reference"=0}, "Grid Descriptor"=T47 {"X Step"=0.3, "Y Step"=0.3, "Unit"=enum."Undefined"}, "Image"=w5142) -> ("Calibrated Image"=→"APD 3":T2)  [unwired: 7 in, 1 out]
      }
    }
    n3593 = case "For computing FFTs for display" shown="True" "Compute FFT" {
      tunnel: w4605 -> [_ w5766]
      frame False {
      }
      frame True {
        n3594 = Build Array("FFT 1 Choice 1", "FFT 1 Choice 2", "FFT 2 Choice 1", "FFT 2 Choice 2") -> (w5759:u16[])
        n3595 = Array Size(array=w5766) -> (size(s)=w5765:i32)
        n3596 = feedback-in #21(w5759) -> ()
        n3597 = feedback #21(u16[] [100, 100, 100, 100]) -> (w5760:u16[])
        n3598 = feedback-in #22("# Spectra to Ave.") -> ()
        n3599 = feedback #22("# Spectra to Ave.") -> (w5757:dbl)
        n3600 = Not Equal?(x="# Spectra to Ave.", y=w5757) -> (x != y?=w5756:bool)
        n3601 = Not Equal?(x=w5759, y=w5760) -> (x != y?=w5758:bool)
        n3602 = feedback #23(1.0) -> (w5743:dbl)
        n3603 = Compound Arithmetic op=OR("Reset FFT", w5758, w5756) -> (w5741:bool)
        n3604 = Select(t=1.0, s=w5741, f=w5743) -> (s? t:f=w5745:dbl)
        n3605 = Greater?(x=w5745, y="# Spectra to Ave.") -> (0:w5764:bool)
        n3606 = Increment(x=w5745) -> (x+1=w5744:dbl)
        n3607 = feedback-in #23(w5744) -> ()
        n3608 = local read "DMA Update Period (s)"() -> (w5739:dbl)
        n3609 = Multiply(x="# Spectra to Ave.", y=w5739) -> (x*y=→"Ave. Time (s)":dbl)
        n3610 = Build Array(cluster{"f0":dbl, "df":dbl, "magnitude":dbl[]} {"f0"=0.0, "df"=0.0, "magnitude"=[]} ("PSD")) -> (w5748:cluster{"f0":dbl, "df":dbl, "magnitude":dbl[]}[])
        n3611 = Build Array(w5748, w5748, w5748, w5748) -> (w5750:T58)
        n3612 = feedback #24(w5750) -> (w5755:T58)
        n3613 = for {
          N: 4 -> [_]
          tunnel: w5759 -> [w5788] mode=indexing
          tunnel: w5766 -> [w5789]
          tunnel: w5765 -> [w5791]
          tunnel: w5741 -> [w5784]
          tunnel: w5764 -> [w5783]
          tunnel: "# Spectra to Ave." -> [w5782]
          tunnel: [w5781] -> w5754 mode=indexing
          tunnel: w5755 -> [w5786] mode=indexing
          tunnel: [w5785] -> w5742 mode=indexing
          tunnel: w5745 -> [w5780]
          n3614 = Less?(x=w5788, y=w5791) -> (x < y?=w5790:bool)
          n3615 = Index Array(array=w5789, index=w5788) -> (element=w5787:waveform(dbl))
          n3616 = case shown="True" w5790 {
            tunnel: w5787 -> [_ w5808]
            tunnel: w5786 -> [w5793 w5806]
            tunnel: [w5793 w5794] -> w5785
            tunnel: w5784 -> [_ w5805]
            tunnel: w5783 -> [_ w5798]
            tunnel: w5782 -> [_ w5797]
            tunnel: [cluster{"f0":dbl, "df":dbl, "magnitude":dbl[]} {"f0"=0.0, "df"=0.0, "magnitude"=[]} ("PSD") w5799] -> w5781
            tunnel: w5780 -> [_ w5796]
            frame False {
            }
            frame True {
              n3617 = call <vilib>:"Std Deviation and Variance.vi"("X"=w5808) -> ("mean"=w5809:dbl)  [unwired: 1 in, 2 out]
              n3618 = Subtract(x=w5808, y=w5809) -> (x-y=w5807:waveform(dbl))
              n3619 = xnode "Spectral Measurements"("Signals"=w5807) -> ("PSD"=w5801:cluster{"f0":dbl, "df":dbl, "magnitude":dbl[]})  [unwired: 1 in, 1 out]
              n3620 = case shown="False" w5805 {
                tunnel: w5806 -> [w5818 _]
                tunnel: [w5814 w5823] -> w5794
                tunnel: w5801 -> [w5817 w5824]
                tunnel: w5798 -> [w5816 _]
                frame False {
                  n3621 = Build Array (concatenate)(w5818, w5817) -> (w5815:cluster{"f0":dbl, "df":dbl, "magnitude":dbl[]}[])
                  n3622 = case shown="True" w5816 {
                    tunnel: w5815 -> [w5819 w5822]
                    tunnel: [w5819 w5820] -> w5814
                    frame False {
                    }
                    frame True {
                      n3623 = Delete From Array(array=w5822, index=0) -> (array with subset deleted=w5820:cluster{"f0":dbl, "df":dbl, "magnitude":dbl[]}[])  [unwired: 1 in, 1 out]
                    }
                  }
                }
                frame True {
                  n3624 = Build Array(w5824) -> (w5823:cluster{"f0":dbl, "df":dbl, "magnitude":dbl[]}[])
                }
              }
              n3625 = for {
                tunnel: w5794 -> [w5813] mode=indexing
                tunnel: [w5812] -> w5804 mode=indexing
                workers-P: _ -> [_]
                n3626 = Unbundle By Name(w5813) -> ("magnitude"=w5812:dbl[])
              }
              n3627 = Transpose 2D Array(2D array=w5804) -> (transposed array=w5803:dbl[][])
              n3628 = for {
                tunnel: w5803 -> [w5811] mode=indexing
                tunnel: [w5810] -> w5802 mode=indexing
                workers-P: _ -> [_]
                n3629 = Add Array Elements(numeric array=w5811) -> (sum=w5810:dbl)
              }
              n3630 = Select(t=w5797, s=w5798, f=w5796) -> (s? t:f=w5795:dbl)
              n3631 = Divide(x=w5802, y=w5795) -> (x/y=w5800:dbl[])
              n3632 = Bundle By Name(cluster=w5801, "magnitude"=w5800) -> (w5799:cluster{"f0":dbl, "df":dbl, "magnitude":dbl[]})
            }
          }
        }
        n3633 = case shown="True" w5741 {
          tunnel: w5742 -> [w5773 w5779]
          tunnel: [w5773 w5774] -> w5740
          frame False {
          }
          frame True {
            n3634 = Array Subset(array=w5779, index (row)=0 ("index"), length (row)=4 ("length"), index (col)=0 ("index"), length (col)=1 ("length")) -> (w5774:T58)
          }
        }
        n3635 = feedback-in #24(w5740) -> ()
        n3636 = Split 1D Array(array=w5754, index=2) -> (first subarray=→"FFT 1":cluster{"f0":dbl, "df":dbl, "magnitude":dbl[]}[], second subarray=→"FFT 2":cluster{"f0":dbl, "df":dbl, "magnitude":dbl[]}[])
      }
    }
    n3637 = local read "T1 calibration"() -> (w4416:T6)
    n3638 = local read "T2 calibration"() -> (w4415:T5)
    n3639 = call-poly <vilib>:"Index Waveform Array.vi"("index"=16, "waveform array"=w4390) -> ("waveform"=w4389:waveform(dbl))  [unwired: 8 in, 1 out]
    n3640 = Unbundle By Name(w4405) -> ("Y"=w4414:dbl[])
    n3641 = Unbundle By Name(w4402) -> ("Y"=w4413:dbl[])
    n3642 = Unbundle By Name(w4389) -> ("Y"=→"PSD Y Sum":dbl[])
    n3643 = call "calibrate trap data.vi"("T2 cal"=w4415, "T2"=w4413, "T1 cal"=w4416, "T1"=w4414) -> ("T2 force (pN)"=w4406:dbl[], "T2 position (nm)"=w4407:dbl[], "T1 force (pN)"=w4408:dbl[], "T1 position (nm)"=w4409:dbl[])
    n3644 = Bundle By Name(cluster=w4405, "Y"=w4409) -> (w4404:waveform(dbl))
    n3645 = Bundle By Name(cluster=w4405, "Y"=w4408) -> (w4403:waveform(dbl))
    n3646 = Bundle By Name(cluster=w4402, "Y"=w4407) -> (w4401:waveform(dbl))
    n3647 = Bundle By Name(cluster=w4402, "Y"=w4406) -> (w4400:waveform(dbl))
    n3648 = Subtract(x=w4409, y=w4407) -> (x-y=w4648:dbl[])
    n3649 = case shown="True" "Read Lateness and Rel Phase" {
      tunnel: w4482 -> [w5070 w5103]
      tunnel: w4481 -> [w5071 w5102]
      tunnel: [w5070 w5075] -> w4646
      tunnel: [w5071 w5074] -> w4645
      frame False {
      }
      frame True {
        n3650 = xnode "Read/Write Control"("FPGA VI Reference In"=w5103, "error in"=w5102) -> ("FPGA VI Reference Out"=w5077:T25, "error out"=w5076:errorcluster, "GI Relative phase"=→"GI relative phase":i16, "Relative phase"=→"Relative phase (AI1)":i16, "AI Late Counter"=→"Late Counter (AI1)":u8, "GI Late Counter"=→"GI Late Counter":u8, "MCL Late Counter"=→"MCL Late Counter":u8, "MCL Relative Phase"=→"Relative Phase (MCL)":i16, "APD Acq Relative Phase"=→"APD Acq Relative Phase":i16, "APD 1 Gate Relative Phase"=→"APD 1 Gate Relative Phase":i16, "APD 2 Gate Relative Phase"=→"APD 2 Gate Relative Phase":i16, "APD Acq Late Counter"=→"APD Acq Late Counter":u8, "APD 1 Gate Late Counter"=→"APD 1 Gate Late Counter":u8, "APD 2 Gate Late Counter"=→"APD 2 Gate Late Counter":u8, "Green FB Relative Phase"=→"Relative phase (Green FB)":i16, "GI Relative phase 2"=→"GI relative phase 2":i16, "GI Late Counter 2"=→"GI Late Counter 2":u8, "Trap Pos FIFO Timeout"=→"Trap Pos FIFO Timeout":u16, "Trap AI FIFO Timeout"=→"Trap AI FIFO Timeout":u16, "RI Late Counter"=→"RI Late Counter":u8, "RI Relative phase"=→"RI relative phase":i16, "Green Late Counter"=→"Green AI Late Counter":u8, "BI Late Counter (AO)"=→"Late Counter (BI AO)":u8, "Blue Late Counter (D)"=→"Late Counter (BI DO)":u8, "BI Relative phase (AO)"=→"Relative phase (BI AO)":i16, "BI Relative phase (D)"=→"Relative phase (BI DO)":i16)
        n3651 = xnode "Read/Write Control"("FPGA VI Reference In"=w5077, "error in"=w5076) -> ("FPGA VI Reference Out"=w5075:T25, "error out"=w5074:errorcluster, "APD 3 Gate Late Counter"=→"APD 3 Gate Late Counter":u8, "APD 3 Gate Relative Phase"=→"APD 3 Gate Relative Phase":i16)
      }
    }
    n3652 = Negate(x=w4648) -> (-x=w4465:dbl[])
    n3653 = Subtract(x=w4465, y="Offset (nm)") -> (x-y=w4622:dbl[])
    n3654 = case "Choose calibrated display" shown="2" "Calibration" {
      tunnel: w4405 -> [w5105 _ _]
      tunnel: w4402 -> [w5104 _ _]
      tunnel: [w5105 w5107 w5109] -> w4661
      tunnel: [w5104 w5106 w5108] -> w4660
      tunnel: w4404 -> [_ w5107 _]
      tunnel: w4403 -> [_ _ w5109]
      tunnel: w4401 -> [_ w5106 _]
      tunnel: w4400 -> [_ _ w5108]
      frame 0, Default {
      }
      frame 1 {
      }
      frame 2 {
      }
    }
    n3655 = Bundle By Name(cluster=w4405, "Y"=w4622) -> (w4399:waveform(dbl))
    "Bead Separation" <- w4399
    n3656 = feedback #25(w4622) -> (w4621:dbl[])
    n3657 = Build Array (concatenate)(w4622, w4621) -> (w4411:dbl[])
    n3658 = Split 1D Array(array=w4411, index=w4525) -> (first subarray=w4412:dbl[])  [unwired: 1 out]
    n3659 = feedback-in #25(w4412) -> ()
    n3660 = Build Array(w4405, w4404, w4403, w4402, w4401, w4400, w4399) -> (w4398:waveform(dbl)[])
    n3661 = Not(x="Trap Trig. Fl.") -> (.not. x?=w4501:bool)
    n3662 = Unbundle By Name(w4661) -> ("Y"=w4466:dbl[])
    n3663 = Unbundle By Name(w4660) -> ("Y"=w4623:dbl[])
    n3664 = call-poly <vilib>:"Mean.vi"("X"=w4412) -> ("mean"=w4618:dbl)  [unwired: 1 out]
    "Bead Mean (nm)" <- w4618
    n3665 = Multiply(x=w4660, y=-1.0) -> (x*y=w4650:waveform(dbl))
    n3666 = call-poly <vilib>:"Mean.vi"("X"=w4466) -> ("mean"=w4469:dbl)  [unwired: 1 out]
    "T1 X" <- w4469
    n3667 = call-poly <vilib>:"Mean.vi"("X"=w4623) -> ("mean"=w4468:dbl)  [unwired: 1 out]
    "T2 X" <- w4468
    n3668 = Build Array(w4661, w4650) -> (→"Force" →"Force 2":waveform(dbl)[])
    n3669 = Subtract(x=w4412, y=w4618) -> (x-y=w4617:dbl[])
    n3670 = Square(x=w4617) -> (x^2=w4616:dbl[])
    n3671 = Negate(x=w4623) -> (-x=w4424:dbl[])
    n3672 = call-poly <vilib>:"Mean.vi"("X"=w4616) -> ("mean"=w4615:dbl)  [unwired: 1 out]
    n3673 = Negate(x=w4468) -> (-x=w4467:dbl)
    n3674 = Square Root(x=w4615) -> (sqrt(x)=w4614:dbl)
    n3675 = Add(x=w4466, y=w4424) -> (x+y=w4624:dbl[])
    n3676 = Add(x=w4469, y=w4467) -> (x+y=w4655:dbl)
    n3677 = Multiply(x=10.0, y=w4614) -> (x*y=→"RMS (Ang)":dbl)
    n3678 = Divide(x=w4624, y=2.0) -> (x/y=w4427:dbl[])
    n3679 = Subtract(x=w4469, y=w4467) -> (x-y=→"Difference":dbl)
    n3680 = Select(t=w4424, s="Only check fixed trap T2", f=w4427) -> (s? t:f=→"Vec Mean of T1 T2":dbl[])
    n3681 = Divide(x=w4655, y=2.0) -> (x/y=w4626:dbl)
    "Mean" <- w4626
    n3682 = feedback-in #26("Trap Trig. Fl.") -> ()
    n3683 = feedback #26("Trap Trig. Fl.") -> (w4499:bool)
    n3684 = And(x=w4501, y=w4499) -> (x .and. y?=w4500:bool)
    n3685 = case "If have just turned off triggering" shown="True" w4500 {
      tunnel: w4482 -> [_ w4905]
      tunnel: w4481 -> [_ w4904]
      frame False {
      }
      frame True {
        w4903 = FALSE ("FPGA Trap Trig")
        n3686 = xnode "Read/Write Control"("FPGA VI Reference In"=w4905, "error in"=w4904, "FPGA Trap Trig"=w4903) -> ("FPGA VI Reference Out"=w4902:T25, "error out"=w4901:errorcluster)
        n3687 = xnode "Read/Write Control"("FPGA VI Reference In"=w4902, "error in"=w4901, "TTrig?"=w4903) -> ()  [unwired: 2 out]
        n3688 = local write "Initializing"(FALSE ("Initializing")) -> ()
        n3689 = local write "Triggered"(FALSE ("Triggered")) -> ()
        n3690 = local write "Waiting"(FALSE ("Waiting")) -> ()
      }
    }
    n3691 = Not(x=w4499) -> (.not. x?=w4512:bool)
    n3692 = And(x="Trap Trig. Fl.", y=w4512) -> (x .and. y?=w4509:bool)
    n3693 = Or(x=w4509, y="Reinitialize") -> (x .or. y?=w4495:bool)
    n3694 = feedback #27(w4505) -> (w4510:string)
    n3695 = Select(t=w4505, s=w4509, f=w4510) -> (s? t:f=w4504:string)
    n3696 = Select(t=w4505, s="Reinitialize", f=w4504) -> (s? t:f=w4503:string)
    n3697 = local read "Tether"() -> (w4627:bool)
    n3698 = feedback #28(0) -> (w4507:i32)
    n3699 = case "For determining if there is a tether still" shown="True" w4627 {
      tunnel: w4626 -> [_ w5029]
      frame False {
      }
      frame True {
        n3700 = Greater?(x="Lost Tether Alarm Threshold (pN)", y=w5029) -> (0:w5027:bool)
        n3701 = case shown="True" w5027 {
          frame False {
          }
          frame True {
            w5030 = FALSE ("Value (Signaling)")
            n3702 = flat-sequence {
              frame #0 {
                # "stop only if saving"
                n3703 = local read "Saving..."() -> (w5042:bool)
                n3704 = And(x=w5042, y="TA Cancel Save?") -> (x .and. y?=w5041:bool)
                n3705 = local write "Stop Saving"(w5041) -> ()
              }
              frame #1 {
                n3706 = case shown="True" "TA Green Off?" {
                  frame False {
                  }
                  frame True {
                    w5045 = FALSE ("Fl. Triggered...")
                    n3707 = local write "Fl. Triggered..."(w5045) -> ()
                    n3708 = property on="Green Laser ON" class="Bool (strict)"("Val(Sgnl)"=w5045) -> ()  [unwired: 2 in, 2 out]
                  }
                }
              }
            }
            n3709 = local read "Time tether formed"() -> (w5036:timestamp)
            n3710 = Get Date/Time In Seconds() -> (seconds since 1Jan1904=w5037:timestamp)
            n3711 = Subtract(x=w5037, y=w5036) -> (x-y=w5035:dbl)
            n3712 = Number To Decimal String(number=w5035) -> (decimal integer string=w5032:string)  [unwired: 1 out]
            n3713 = local read "Messages"() -> (w5039:string)
            n3714 = call <vilib>:"Beep.vi"() -> ()  [unwired: 3 in, 9 out]
